vi "gfitsio-scan-date-time-string.vi"(8 "error in (no error)":errorcluster, 11 "date/time string":string) -> (0 "error out":errorcluster, 2 "timestamp":timestamp)   [LabVIEW 2011, in "gfitsio.lvlib"]
doc: "Parses a LabVIEW timestamp value from a 23 character date-time string using the following format: YYYY-MM-DDTHH:MM:SS.SSS where\n\nYYYY -- Four digit year\nMM -- Two digit month\nDD -- Two digit day of month\nT -- Literal separator\nHH -- Two digit hour using 24-hour format\nMM -- Two digit minute\nSS.SSS -- Two digit seconds to millisecond precision"
uses:
  gfitsio.lvlib
panel:
  in  "for type":T1
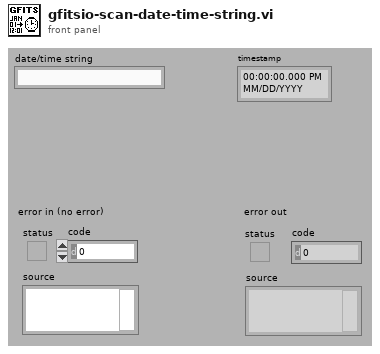
[diagram p1: front panel]
types:
  T1 = cluster{"second":i32, "minute":i32, "hour":i32, "day of month":i32, "month":i32, "year":i32, "day of week":i32, "day of year":i32, "is DST":i32}
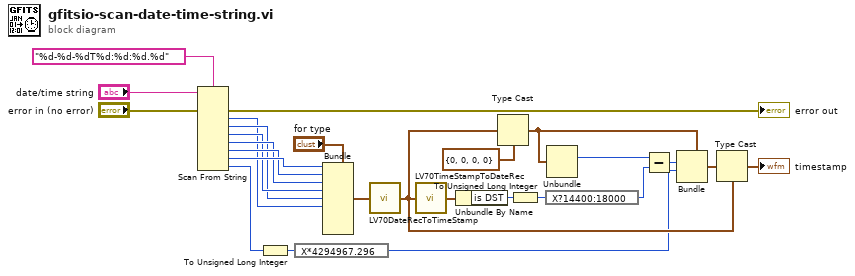
[diagram p0: block diagram]
diagram:
  n1 = Scan From String(format string="%d-%d-%dT%d:%d:%d.%d", input string="date/time string", error in="error in (no error)") -> (error out=→"error out":errorcluster, output 1=w19:i32, output 2=w20:i32, output 3=w21:i32, output 4=w22:i32, output 5=w23:i32, output 6=w24:i32, output 7=w25:i32)  [unwired: 8 in, 2 out]
  n2 = To Unsigned Long Integer(number=w25) -> (unsigned 32bit integer=w4:u32)
  n3 = expression code="X*4294967.296"(w4) -> (w5:u32)
  n4 = Bundle(cluster="for type", "second"=w24, "minute"=w23, "hour"=w22, "day of month"=w21, "month"=w20, "year"=w19) -> (w8:T1)  [unwired: 3 in]
  n5 = call <vilib>:"LV70DateRecToTimeStamp.vi"("date time rec"=w8) -> ("Time Stamp"=w6:timestamp)
  n6 = call <vilib>:"LV70TimeStampToDateRec.vi"("time stamp"=w6) -> ("date time rec"=w7:T1)
  n7 = Unbundle By Name(w7) -> ("is DST"=w17:i32)
  n8 = Type Cast(type=cluster{u32, u32, u32, u32} {0, 0, 0, 0}, x=w6) -> (*(type *) &x=w12:cluster{u32, u32, u32, u32})
  n9 = To Unsigned Long Integer(number=w17) -> (unsigned 32bit integer=w13:u32)
  n10 = expression code="X?14400:18000"(w13) -> (w14:u32)
  n11 = Unbundle(w12) -> (w15:u32)  [unwired: 3 out]
  n12 = Subtract(x=w15, y=w14) -> (x-y=w11:u32)
  n13 = Bundle(cluster=w12, w11, w5) -> (w10:cluster{u32, u32, u32, u32})  [unwired: 2 in]
  n14 = Type Cast(type=w6, x=w10) -> (*(type *) &x=→"timestamp":timestamp)
